vi "Tach Process Analog (Export State).vi"(0 "input signal":sgl[](array[numeric]), 1 "sampling rate [Hz]":dbl=5120.0, 2 "reset? (F)":bool, 5 "PPR":dbl, 7 "Thresh(V)":dbl, 9 "Slope":u16, 11 "hysteresis (0)":dbl format="%.2f", 12 "pulse width (2)":i32=2, 13 "state in":T1) -> (4 "speed position info":T2, 6 "binary tach signal":sgl[](array[numeric]), 14 "state out":T1)   [LabVIEW 2017, in "VibrationAnalysisFunctions.lvlib"]
doc: "Locates tachometer pulse positions in analog tachometer signals. The data type you wire to the <B>analog tacho signal</B> input determines the polymorphic instance to use."
uses:
  <vilib>/addons/InsightCM/Utilities/Analysis/Vibration/VibrationAnalysisFunctions.lvlib
  <vilib>/addons/Sound and Vibration/Order Analysis/Misc/OAT Position Info.ctl
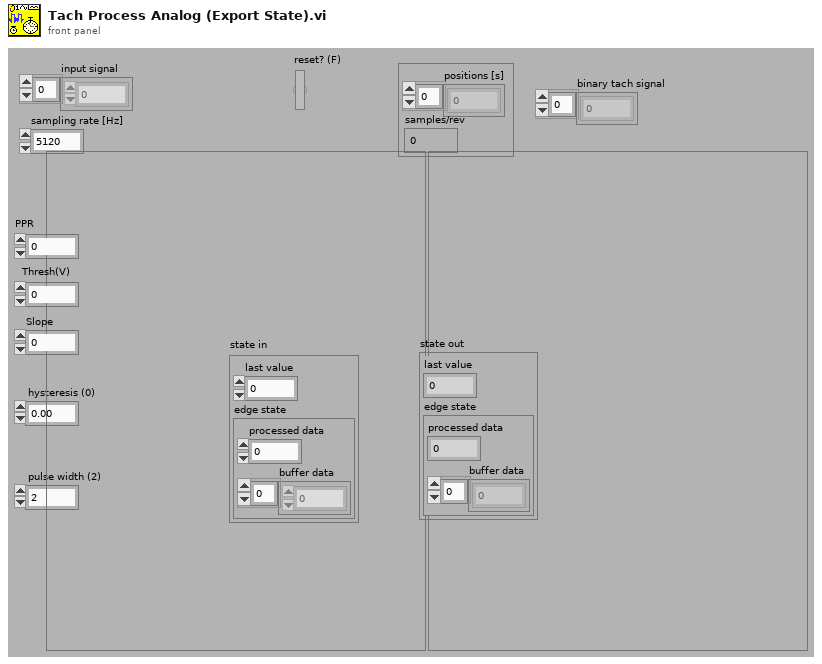
[diagram p1: front panel]
types:
  T1 = cluster{"last value":dbl, "edge state":cluster{"processed data":dbl, "buffer data":dbl[]}}
  T2 = typedef "OAT Position Info.ctl" = cluster{"positions [s]":dbl[], "samples/rev":dbl}
  T3 = cluster{"processed data":dbl, "buffer data":dbl[]}
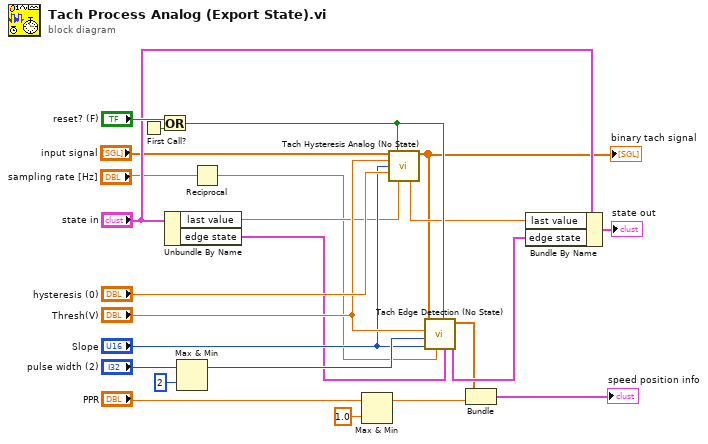
[diagram p0: block diagram]
diagram:
  n1 = First Call?() -> (First Call?: T/F=w23:bool)
  n2 = Or(x="reset? (F)", y=w23) -> (x .or. y?=w18:bool)
  n3 = Unbundle By Name("state in") -> ("last value"=w13:dbl, "edge state"=w12:T3)
  n4 = Max & Min(x="pulse width (2)", y=2) -> (max(x,y)=w21:i32)  [unwired: 1 out]
  n5 = Reciprocal(x="sampling rate [Hz]") -> (1/x=w1:dbl)
  n6 = Max & Min(x="PPR", y=1.0) -> (max(x,y)=w3:dbl)  [unwired: 1 out]
  n7 = call <vilib>:"Tach Hysteresis Analog (No State).vi"("input signal"="input signal", "reset? (T)"=w18, "threshold (auto)"="Thresh(V)", "slope (Rising)"="Slope", "hysteresis(0)"="hysteresis (0)", "last value in"=w13) -> ("output signal"=w6:sgl[], "last value out"=w11:sgl)  [unwired: 7 in, 1 out]
  "binary tach signal" <- w6
  n8 = call <vilib>:"Tach Edge Detection (No State).vi"("state in"=w12, "reset? (True)"=w18, "dt"=w1, "slope (Rising)"="Slope", "pulse width (2)"=w21, "threshold (0.0)"="Thresh(V)", "x[n]"=w6) -> ("state out"=w10:T3, "pulse positions [s]"=w5:dbl[])  [unwired: 3 in]
  n9 = Bundle("pulse positions [s]"=w5, w3) -> (→"speed position info":cluster{"pulse positions [s]":dbl[], dbl})  [unwired: 1 in]
  n10 = Bundle By Name(cluster="state in", "last value"=w11, "edge state"=w10) -> (→"state out":T1)
